vi "CryoCooler_AVC_Serial_Write_and_Read_fast.vi"(8 "error in (no error)":errorcluster, 9 "Command Options":string, 10 "Command":T1 items=["STATUS", "COOLER", "E", "ERROR", "KD", "KI", "KP", "LOGIN", "LOGOUT", "MODE", "P", "PWOUT", "SENSOR", "TC", "TEMP RJ", "TTARGET", "VERSION"], 11 "VISA Resource (write)":refnum<visa-resource-name>="COM1") -> (0 "error out":errorcluster, 2 "VISA Resource out":refnum<visa-resource-name>="COM1", 3 "read string array":string[](array[string]))   [LabVIEW 2021]
doc: "This example opens two VISA resources and configures one COM port to perform a write operation and the other COM port to perform a read operation. This VI will wait until the specified number of bytes is received at the port or until a termination character is read.\n\nThis example allows you perform diagnostic tests on your ports. You can use this example to perform a wrap-back test. Both serial ports must have the same basic configuration parameters. You can connect two of the ports using a null modem cable, which effectively connects one port's RX lines to the other port's TX lines. If you use a straight-through cable, one port's RX lines will be connected to the other port's RX lines, and you cannot communicate between the two ports."
uses:
  Cryo Cooler/CryoCoolerAVC/CryoCoolerAVC Command enum.ctl
panel:
  in  "Custom Command":string
  out "bytes read array":u32[](array[numeric])
  out "Read String":string
  out "bytes read":u32
  out "bytes written":u32
  in  "Tab Control":enum32{"Standard command", "Custom command"}(tab)
  in  "Lines to read":u16
  # "Overview: Demonstrates the use of the VISA functions to communicate between two different serial devices.\nRequirements: NI-VISA Driver, two serial devices\nInstructions:\n1. Ensure the resources specified by VISA Resource (write) and VISA Resource (read) are valid serial devices.\n2. Connect a null modem RS-232 or RS-485/422 cable between the 2 ports.\n3. Run the VI.\n4. If your two devices are connected properly, you should see the Read String value match the Write String value."
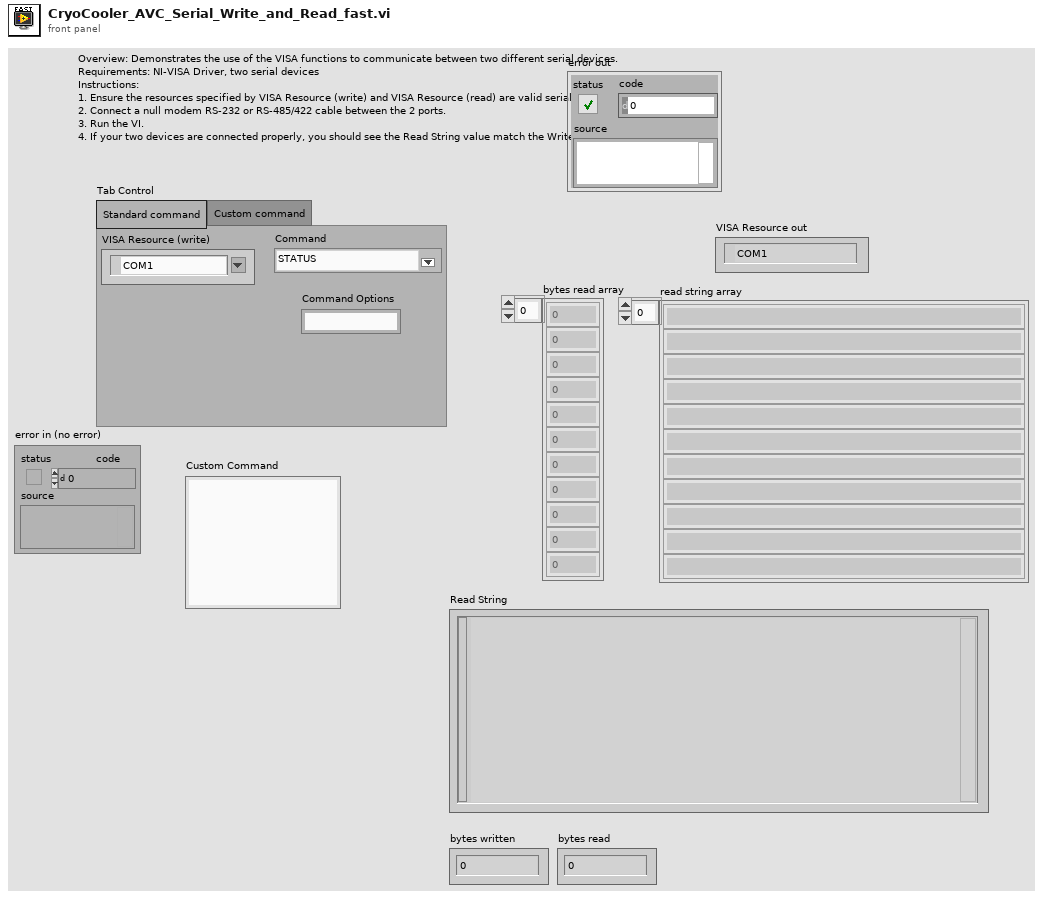
[diagram p1: front panel]
types:
  T1 = typedef "CryoCoolerAVC Command enum.ctl" = u16
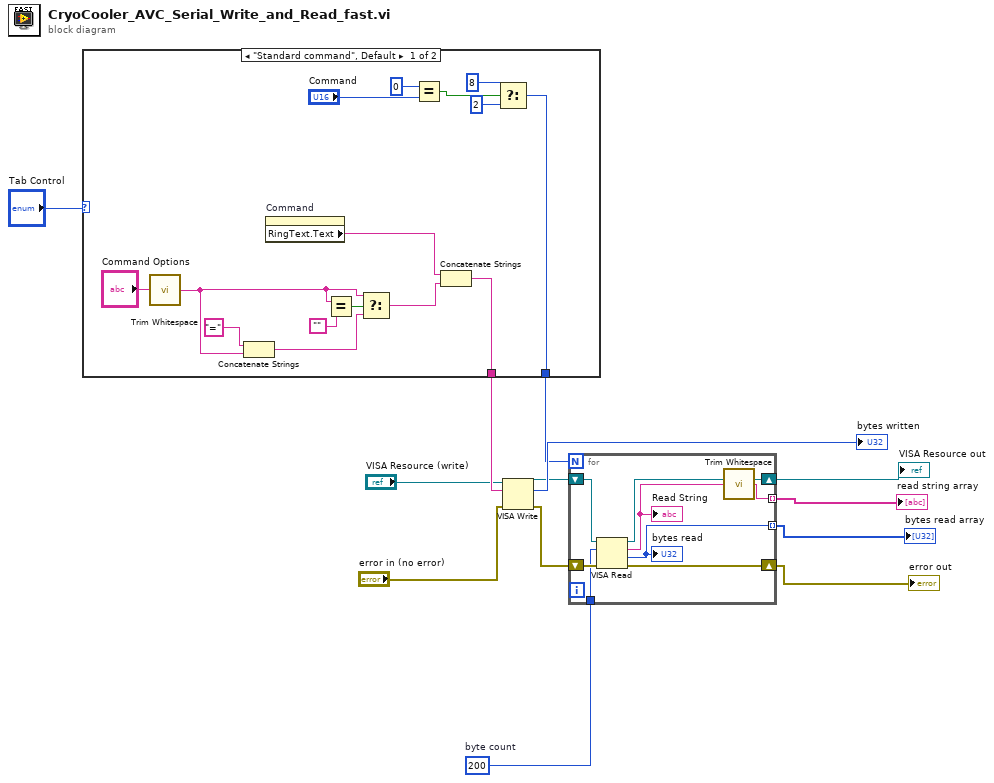
[diagram p0: block diagram]
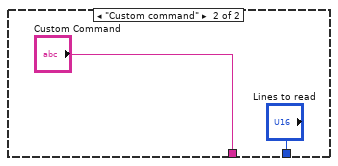
[diagram p2: hidden frame]
diagram:
  w9 = u32 200  # byte count
  n1 = case shown="\"Standard command\", Default" "Tab Control" {
    tunnel: [w23 "Lines to read"] -> w8
    tunnel: [w14 "Custom Command"] -> w7
    frame "Standard command", Default {
      n2 = call <vilib>:"Trim Whitespace.vi"("string"="Command Options") -> ("trimmed string"=w18:string)  [unwired: 1 in]
      n3 = Concatenate Strings("=" ("string"), w18) -> (w19:string)
      n4 = property on="Command" class="Ring (strict)"() -> ("RingText.Text"=w15:string)  [unwired: 2 in, 2 out]
      n5 = Equal?(x=w18, y="") -> (x = y?=w20:bool)
      n6 = Select(t=w18, s=w20, f=w19) -> (s? t:f=w16:string)
      n7 = Equal?(x=u16 0, y="Command") -> (x = y?=w26:bool)
      n8 = Concatenate Strings(w15, w16) -> (w14:string)
      n9 = Select(t=u16 8 ("x"), s=w26, f=u16 2) -> (s? t:f=w23:u16)
    }
    frame "Custom command" {
    }
  }
  n10 = VISA Write(VISA resource name="VISA Resource (write)", write buffer=w7, error in (no error)="error in (no error)") -> (VISA resource name out=w1:refnum<visa-resource-name>, return count=→"bytes written":u32, error out=w12:errorcluster)
  n11 = for {
    N: w8 -> [_]
    tunnel: [w31] -> w11 mode=indexing
    shift-right: [w37] -> w5
    shift-left: w1 -> [w38]
    shift-right: [w35] -> w2
    shift-left: w12 -> [w36]
    tunnel: [w33] -> w10 mode=indexing
    tunnel: w9 -> [w32]
    n12 = VISA Read(VISA resource name=w38, byte count=w32, error in (no error)=w36) -> (VISA resource name out=w37:refnum<visa-resource-name>, read buffer=w34:string, return count=w33:u32, error out=w35:errorcluster)
    "Read String" <- w34
    "bytes read" <- w33
    n13 = call <vilib>:"Trim Whitespace.vi"("string"=w34) -> ("trimmed string"=w31:string)  [unwired: 1 in]
  }
  "read string array" <- w11
  "bytes read array" <- w10
  "VISA Resource out" <- w5
  "error out" <- w2
